vi "Get_Att_Value.vi"(8 "error in (no error)":errorcluster, 11 ".NET Reference in":refnum<k24>) -> (0 "error out":errorcluster, 2 "att out":dbl, 3 "Reference out":refnum<k24>)   [LabVIEW 2017]
uses:
  LV_IL_Sample/DLL/InstrumentDLL.dll
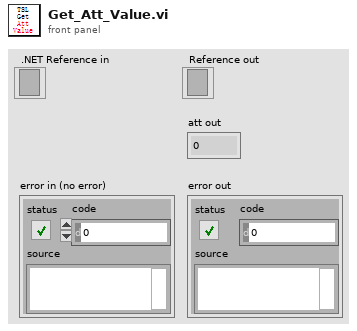
[diagram p1: front panel]
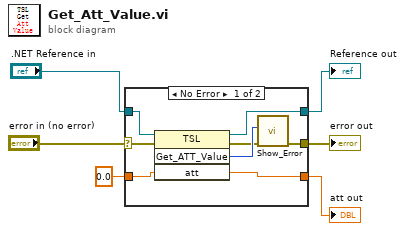
[diagram p0: block diagram]
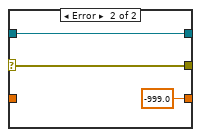
[diagram p2: hidden frame]
diagram:
  n1 = case shown="No Error" "error in (no error)" {
    selector: "error in (no error)" -> [w7 w17]
    tunnel: [w14 -999.0 ("att")] -> w6
    tunnel: ".NET Reference in" -> [w13 w16]
    tunnel: [w12 w16] -> w4
    tunnel: [w8 w17] -> w3
    tunnel: 0.0 ("att") -> [w11 _]
    frame No Error {
      n2 = invoke on="调用节点" class="TSL" method="Get_ATT_Value"(reference=w13, error in=w7, "att"=w11) -> (reference out=w12:refnum<k24>, error out=w9:errorcluster, "Get_ATT_Value"=w10:i32, "att"=w14:dbl)  [unwired: 1 in]
      n3 = call "Show_Error.vi"("error in (no error)"=w9, "Error"=w10) -> ("error out"=w8:errorcluster)  [unwired: 9 in]
    }
    frame Error {
    }
  }
  "att out" <- w6
  "Reference out" <- w4
  "error out" <- w3
